vi "CTR_ReaderWriter-EndpointURL.vi"(8 "DAQ ID #":i32, 9 "CTR Endpoint":string, 10 "DAQ IR Addr":string, 11 "CTR IP Addr":string) -> (0 "CTR Endpoint":string="CTR001", 1 "DAQ Endpoint":string, 2 "DAQ URL":string, 3 "CTR URL":string)   [LabVIEW 2024]
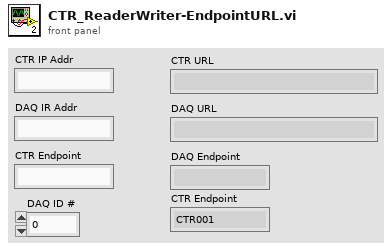
[diagram p1: front panel]
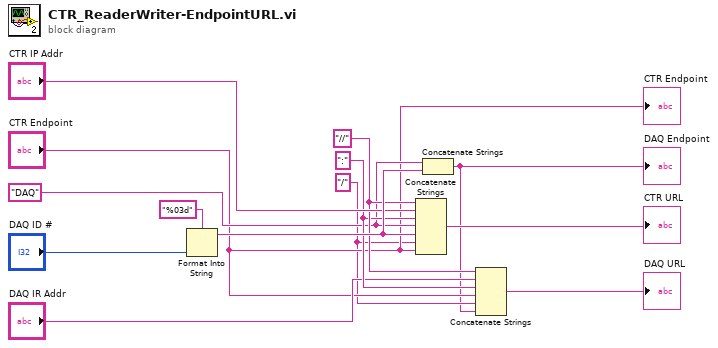
[diagram p0: block diagram]
diagram:
  w5 = "DAQ" ("string")
  w6 = ":" ("string")
  w7 = "//" ("string")
  w2 = "/" ("string")
  n1 = Format Into String(format string="%03d", "DAQ ID #") -> (resulting string=w13:string)  [unwired: 2 in, 1 out]
  n2 = Concatenate Strings(w7, "CTR IP Addr", w6, w5, w13, w2, "CTR Endpoint") -> (→"CTR URL":string)
  n3 = Concatenate Strings(w5, w13) -> (w1:string)
  "DAQ Endpoint" <- w1
  n4 = Concatenate Strings(w7, "DAQ IR Addr", w6, "CTR Endpoint", w2, w1) -> (→"DAQ URL":string)
  "CTR Endpoint" <- "CTR Endpoint"
